vi "Choose Color.vi"(8 "error in (no error)":errorcluster, 10 "NamedColors":T1=enum."WhiteSmoke", 11 "Color in":refnum<class "Color.lvclass">) -> (0 "error out":errorcluster, 3 "Color out":refnum<class "Color.lvclass">)   [LabVIEW 2014, in "DataGrid.lvlib" / "Color.lvclass"]
doc: "Picks a color from a list of known names and stores the corresponding color in the color class for use with .net objects."
uses:
  Color.lvclass
  NamedColors.ctl
  Color.lvclass/Color.ctl
  System.Drawing
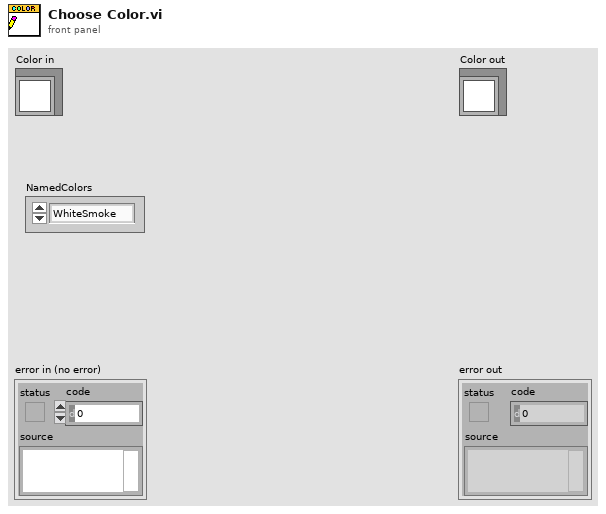
[diagram p1: front panel]
types:
  T1 = typedef "DataGrid.lvlib/Color.lvclass/NamedColors.ctl" = enum16{"AliceBlue", "AntiqueWhite", "Aqua", "Aquamarine", "Azure", "Beige", "Bisque", "Black", "BlanchedAlmond", "Blue", "BlueVilot", "Brown", "BurlyWood", "CadetBlue", "Chartreuse", "Chocolate", "Coral", "CornflowerBlue", "Cornsilk", "Crimson", "Cyan", "DarkBlue", "DarkCyan", "DarkGoldenrod", "DarkGray", "DarkGreen", "DarkKhaki", "DarkMagenta", "DarkOliveGreen", "DarkOrange", "DarkOrchid", "DarkRed", "DarkSalmon", "DarkSeaGreen", "DarkSlateBlue", "DarkSlateGray", "DarkTurquoise", "DarkViolet", "DeepPink", "DeepSkyBlue", "DimGraw", "DodgerBlue", "Firebrick", "FlaralWhite", "ForestGreen", "Fuchsia", "Gainsboro", "GhostWhite", "Gold", "Goldenrod", "Gray", "Green", "GreenYellow", "Honeydew", "HotPink", "IndianRed", "Indigo", "Ivory", "Khaki", "Lavender", "LavenderBlush", "LawnGreen", "LemonChiffon", "LightBlue", "LightCoral", "LightCyan", "LightGoldenrodYellow", "LightGray", "LightGreen", "LightPink", "LightSalmon", "LightSeaGreen", "LightSkyBlue", "LightSlateGray", "LightSteelBlue", "LightYellow", "Lime", "LimeGreen", "Linen", "Magenta", "Maroon", "MediumAquamarine", "MediumBlue", "MediumOrchid", "MediumPurple", "MediumSeaGreen", "MediumSlateBlue", "MediumSpringGreen", "MediumTurquoise", "MediumVioletRed", "MidnightBlue", "MintCream", "MistyRose", "Moccasin", "MavajoWhite", "Navy", "OldLave", "Olive", "OliveDrab", "Orange", "OrangeRed", "Orchid", "PaleGoldenrod", "PaleGreen", "PaleTurquoise", "PaleViloetRed", "PapayaWhip", "PeachPuff", "Peru", "Pink", "Plum", "PowerBlue", "Purple", "Red", "RosyBrown", "RoyalBlue", "SaddleBrown", "Salmon", "SandyBrown", "SeaGreen", "SeaShell", "Sienna", "Silver", "SkyBlue", "SlateBlue", "SlateGray", "Snow", "SpringGreen", "SteelBlue", "Tan", "Teal", "Thistle", "Tomato", "Transparent", "Turquoise", "Violet", "Wheat", "White", "WhiteSmoke", "Yellow", "YellowGreen"}
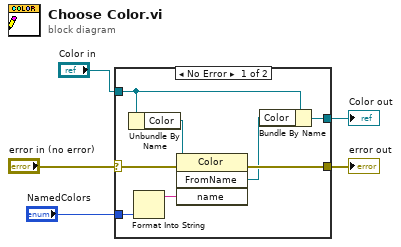
[diagram p0: block diagram]
diagram:
  n1 = case shown="No Error" "error in (no error)" {
    selector: "error in (no error)" -> [w12 w14]
    tunnel: [w11 w14] -> w4
    tunnel: [w13 w15] -> w2
    tunnel: "Color in" -> [w8 w15]
    tunnel: "NamedColors" -> [w10 _]
    frame No Error {
      n2 = Unbundle By Name(w8) -> ("Color"=w7:refnum<k24>)
      n3 = Format Into String(w10) -> (resulting string=w9:string)  [unwired: 3 in, 1 out]
      n4 = invoke class="Color" method="FromName"(reference=w7, error in=w12, "name"=w9) -> (error out=w11:errorcluster, "FromName"=w6:refnum<k24>)  [unwired: 1 in, 2 out]
      n5 = Bundle By Name(cluster=w8, "Color"=w6) -> (w13:refnum<class "Color.lvclass">)
    }
    frame Error {
    }
  }
  "error out" <- w4
  "Color out" <- w2
